vi "Read VI name.vi"(9 "SubVI in":refnum<class "SubVI.lvclass">) -> (3 "SubVI out":refnum<class "SubVI.lvclass">, 4 "VI name":string)   [LabVIEW 2014]
uses:
  SubVI.lvclass
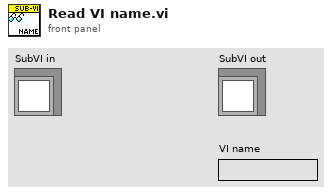
[diagram p1: front panel]
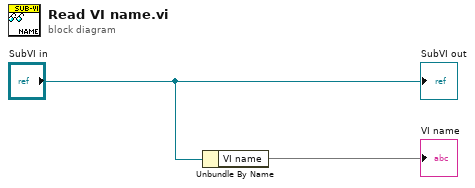
[diagram p0: block diagram]
diagram:
  n1 = Unbundle By Name("SubVI in") -> ("VI name"=→"VI name")
  "SubVI out" <- "SubVI in"
